vi "button.vi"(1 "Down":bool, 2 "Up":bool) -> (0 "Elevator Request":dbl)   [LabVIEW 2014]
panel:
  out "Requested Level":dbl
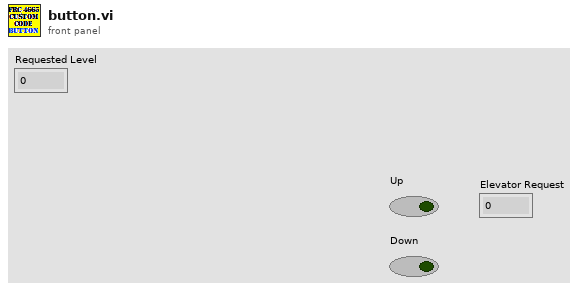
[diagram p1: front panel]
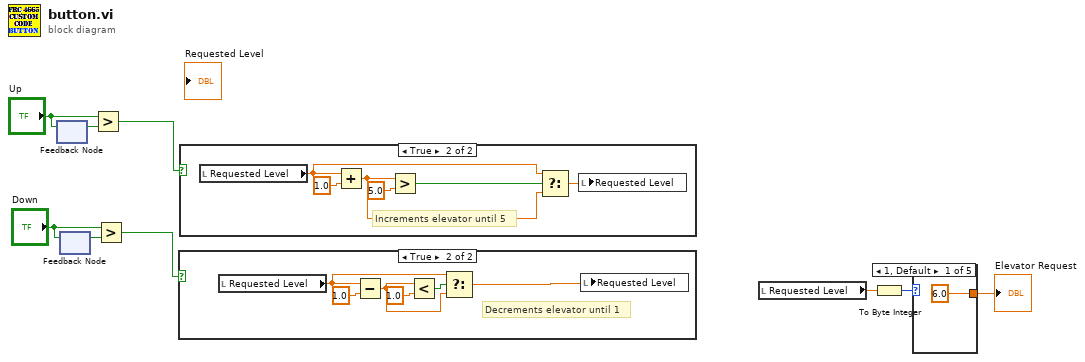
[diagram p0: block diagram]
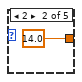
[diagram p2: hidden frame]
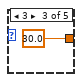
[diagram p3: hidden frame]
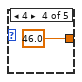
[diagram p4: hidden frame]
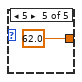
[diagram p5: hidden frame]
diagram:
  n1 = feedback #1() -> (w9:bool)  [unwired: 1 in]
  n2 = feedback-in #1("Up") -> ()
  n3 = feedback #2() -> (w7:bool)  [unwired: 1 in]
  n4 = feedback-in #2("Down") -> ()
  n5 = Greater?(x="Up", y=w9) -> (0:w8:bool)
  n6 = Greater?(x="Down", y=w7) -> (0:w6:bool)
  n7 = case shown="True" w6 {
    frame False {
    }
    frame True {
      # "Decrements elevator until 1"
      n8 = local read "Requested Level"() -> (w11:dbl)
      n9 = Subtract(x=w11, y=1.0) -> (x-y=w13:dbl)
      n10 = Less?(x=w13, y=1.0) -> (x < y?=w14:bool)
      n11 = Select(t=w11, s=w14, f=w13) -> (s? t:f=w10:dbl)
      n12 = local write "Requested Level"(w10) -> ()
    }
  }
  n13 = case shown="True" w8 {
    frame False {
    }
    frame True {
      # "Increments elevator until 5"
      n14 = local read "Requested Level"() -> (w17:dbl)
      n15 = Add(x=w17, y=1.0) -> (x+y=w18:dbl)
      n16 = Greater?(x=w18, y=5.0) -> (0:w19:bool)
      n17 = Select(t=w17, s=w19, f=w18) -> (s? t:f=w16:dbl)
      n18 = local write "Requested Level"(w16) -> ()
    }
  }
  n19 = local read "Requested Level"() -> (w4:dbl)
  n20 = To Byte Integer(number=w4) -> (8bit integer=w5:i8)
  n21 = case shown="1, Default" w5 {
    tunnel: [6.0 ("Elevator Req 2") 14.0 ("Elevator Req 2") 30.0 ("Elevator Req 2") 46.0 ("Elevator Req 2") 62.0 ("Elevator Req 2")] -> w3
    frame 1, Default {
    }
    frame 2 {
    }
    frame 3 {
    }
    frame 4 {
    }
    frame 5 {
    }
  }
  "Elevator Request" <- w3
